vi "PMI.vi"(0 "System no.":i32=1 min=1 max=4 step=1, 2 "Affected axes":string[](array[string]), 3 "Negative limit":dbl[](array[numeric]) format="%.6f", 4 "No.of digits":i16=4, 5 "error in":errorcluster) -> (19 "error out":errorcluster)   [LabVIEW 2020]
doc: "Sets the minimum position limit for specified axes. No. of digits is the number of digits after the decimal point in the limit values that will be sent. Old command-please use NLM if the system supports that command."
panel:
  # "Sets the minimum position limit for specified axes. (new: NLM)"
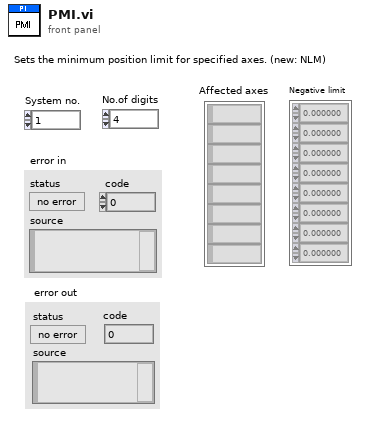
[diagram p1: front panel]
types:
  T1 = enum16{"Disable error check", "Force error check", "Use global settings"}
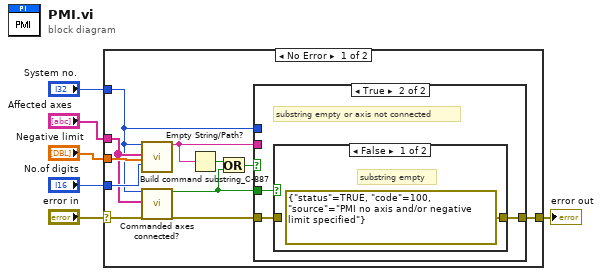
[diagram p0: block diagram]
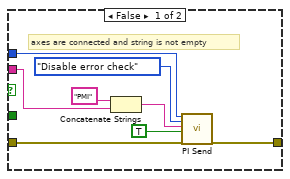
[diagram p2: hidden frame]
diagram:
  n1 = case shown="No Error" "error in" {
    selector: "error in" -> [w11 w31]
    tunnel: [w17 w31] -> w6
    tunnel: "Negative limit" -> [w16 _]
    tunnel: "No.of digits" -> [w15 _]
    tunnel: "System no." -> [w12 _]
    tunnel: "Affected axes" -> [w13 _]
    frame No Error {
      n2 = call "Build command substring_C-887.vi"("System no."=w12, "Affected axes"=w13, "Parameters"=w16, "No. of digits"=w15) -> ("Command substring"=w10:string)  [unwired: 3 in, 12 out]
      n3 = call "Commanded axes connected?.vi"("System no."=w12, "Commanded axes"=w13, "error in"=w11) -> ("Controller error"=w8:bool, "error out"=w14:errorcluster)  [unwired: 1 in, 14 out]
      n4 = Empty String/Path?(string/path=w10) -> (empty?=w9:bool)
      n5 = Or(x=w9, y=w8) -> (x .or. y?=w7:bool)
      n6 = case shown="True" w7 {
        tunnel: w10 -> [w24 _]
        tunnel: [w20 w28] -> w17
        tunnel: w14 -> [w21 w26]
        tunnel: w8 -> [_ w27]
        tunnel: w12 -> [w19 _]
        frame False {
          # "axes are connected and string is not empty"
          n7 = Concatenate Strings("PMI", w24) -> (w22:string)
          n8 = call "PI Send.vi"("System no."=w19, "Error check settings"=T1."Disable error check", "String to send"=w22, "Attach termination char.?"=TRUE ("Attach Linefeed?"), "error in"=w21) -> ("error out"=w20:errorcluster)  [unwired: 1 in, 13 out]
        }
        frame True {
          # "substring empty or axis not connected"
          n9 = case shown="False" w27 {
            tunnel: [errorcluster {"status"=TRUE, "code"=100, "source"="PMI no axis and/or negative limit specified"} ("error out") w30] -> w28
            tunnel: w26 -> [_ w30]
            frame False {
              # "substring empty"
            }
            frame True {
              # "commanded axis not connected"
            }
          }
        }
      }
    }
    frame Error {
    }
  }
  "error out" <- w6
